vi "Enqueue Read.vi"(8 "Error In":errorcluster, 10 "Message":string="Open Connection", 11 "Name":string) -> (0 "Error Out":errorcluster, 2 "Data":variant)   [LabVIEW 2019, in "Kolmogan Library 1.lvlib"]
uses:
  Kolmogan Library 1.lvlib
  Data Error Notifier/Data and Error Notifier.lvlib
  Queue/Queue.lvlib
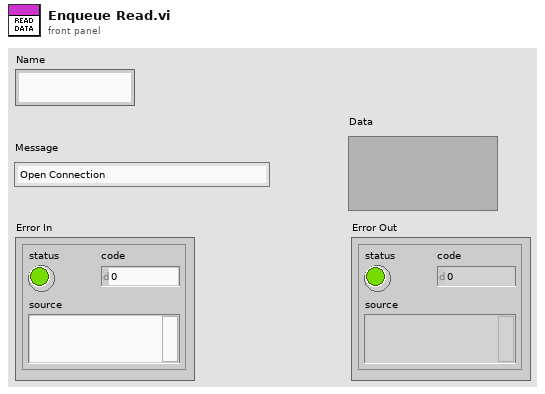
[diagram p1: front panel]
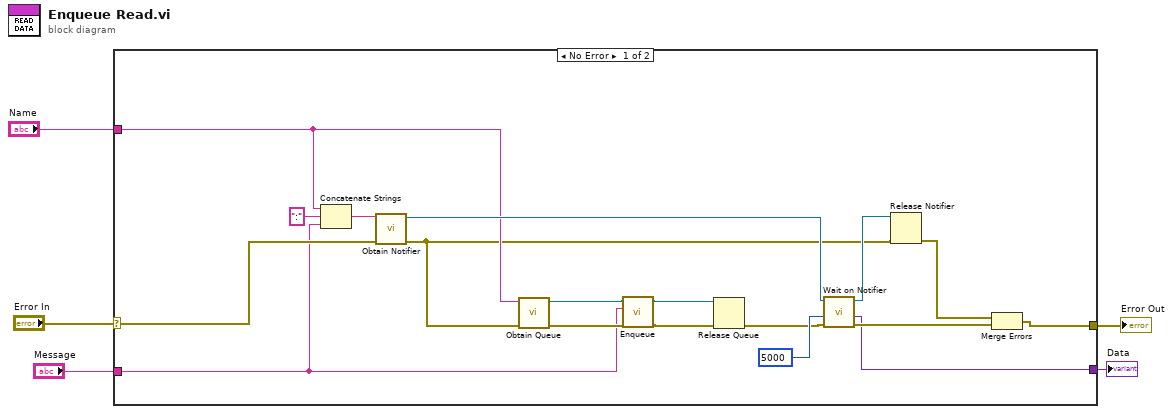
[diagram p0: block diagram]
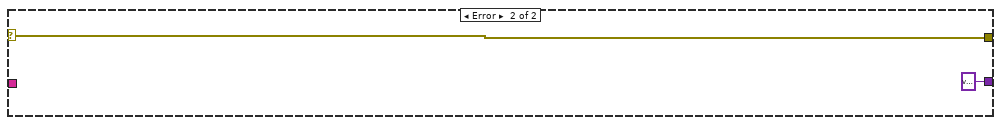
[diagram p2: hidden frame]
diagram:
  n1 = case shown="No Error" "Error In" {
    selector: "Error In" -> [w19 w25]
    tunnel: [w21 w25] -> w4
    tunnel: "Name" -> [w13 _]
    tunnel: "Message" -> [w7 _]
    tunnel: [w6 variant ("Data")] -> w1
    frame No Error {
      n2 = Concatenate Strings(w13, ":" ("string"), w7) -> (w20:string)
      n3 = call "Obtain Notifier.vi"("Error In"=w19, "Name"=w20) -> ("Error Out"=w12:errorcluster, "notifier out"=w14:refnum<notifier>)  [unwired: 8 in]
      n4 = call "Obtain Queue.vi"("Error In"=w12, "Name"=w13) -> ("Error Out"=w8:errorcluster, "queue out"=w11:refnum<queue>)  [unwired: 8 in]
      n5 = call "Enqueue.vi"("Error In"=w8, "Message"=w7, "queue in"=w11) -> ("Error Out"=w10:errorcluster, "queue out"=w9:refnum<queue>)  [unwired: 7 in]
      n6 = Release Queue(queue=w9, error in (no error)=w10) -> (error out=w15:errorcluster)  [unwired: 1 in, 2 out]
      n7 = call "Wait on Notifier.vi"("Error In"=w15, "timeout in ms (-1)"=5000, "notifier in"=w14) -> ("Error Out"=w17:errorcluster, "Data"=w6:variant, "notifier out"=w18:refnum<notifier>)  [unwired: 6 in]
      n8 = Release Notifier(notifier=w18, error in (no error)=w12) -> (error out=w22:errorcluster)  [unwired: 1 in, 2 out]
      n9 = Merge Errors(w22, w17) -> (w21:errorcluster)
    }
    frame Error {
    }
  }
  "Error Out" <- w4
  "Data" <- w1
